vi "ThicknessToPosition.vi"(11 "Thickness":dbl) -> (3 "Position":dbl)   [LabVIEW 2013]
uses:
  Global.vi
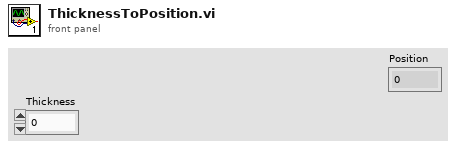
[diagram p1: front panel]
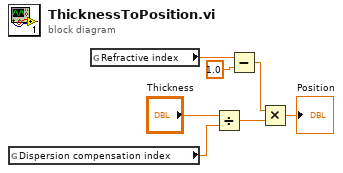
[diagram p0: block diagram]
diagram:
  n1 = global read "Global.vi" "Dispersion compensation index"() -> (w1:dbl)
  n2 = global read "Global.vi" "Refractive index"() -> (w2:dbl)
  n3 = Divide(x="Thickness", y=w1) -> (x/y=w3:dbl)
  n4 = Subtract(x=w2, y=1.0) -> (x-y=w6:dbl)
  n5 = Multiply(x=w6, y=w3) -> (x*y=→"Position":dbl)
